vi "ColorizeREPL.vi"(0 "Data In":T1={"VISA Refnum in"="", "Python Code"="Hi"}, 2 "refs":cluster{"Code":refnum<vi>, "Panel":refnum<vi>}, 4 "Add Spaces?":bool) -> (7 "Data out":T1={"VISA Refnum in"="", "Python Code"="Hi"})   [LabVIEW 2016]
uses:
  <vilib>/Utility/miscctls.llb/LVSelectionTypeDef.ctl
  uPythonX/PythonData.ctl
  uPythonX/uPythonX.xctl
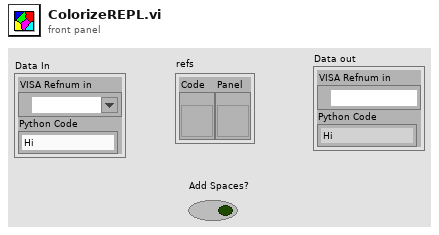
[diagram p1: front panel]
types:
  T1 = typedef "uPythonX.xctl/PythonData.ctl" = cluster{"VISA Refnum in":refnum<visa-resource-name>, "Python Code":string}
  T2 = typedef "LVSelectionTypeDef.ctl" = cluster{"Selection Start":u32, "Selection End":u32}
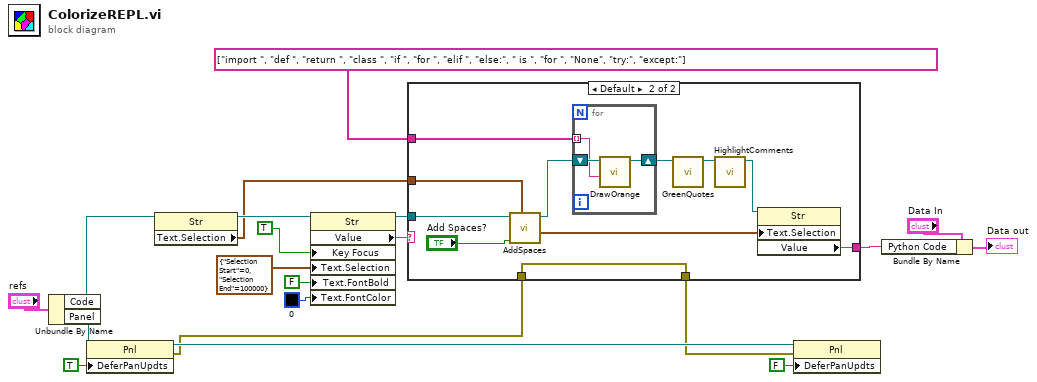
[diagram p0: block diagram]
diagram:
  n1 = Unbundle By Name("refs") -> ("Code"=w3:refnum<vi>, "Panel"=w4:refnum<vi>)
  n2 = property class="Pnl"(reference=w4, "DeferPanUpdts"=TRUE ("Defer Panel Updates")) -> (reference out=w6:refnum<vi>, error out=w1:errorcluster)  [unwired: 1 in]
  n3 = property on="Property Node" class="Str"(reference=w3) -> (reference out=w16:refnum<vi>, "Text.Selection"=w15:T2)  [unwired: 1 in, 1 out]
  n4 = property on="Property Node" class="Str"(reference=w16, "Key Focus"=TRUE, "Text.Selection"=T2 {"Selection Start"=0, "Selection End"=100000}, "Text.FontBold"=FALSE ("Text.Font:Bold"), "Text.FontColor"=u32 0) -> (reference out=w14:refnum<vi>, "Value"=w13:string)  [unwired: 1 in, 1 out]
  n5 = case shown="Default" w13 {
    selector: w13 -> [w22 _]
    tunnel: w14 -> [_ w27]
    tunnel: w15 -> [_ w32]
    tunnel: [w22 w30] -> w10
    tunnel: string[] ["import ", "def ", "return ", "class ", "if ", "for ", "elif ", "else:", " is ", "for ", "None", "try:", "except:"] -> [_ w25]
    tunnel: [w21 w23] -> w2
    tunnel: w1 -> [w21 w23]
    frame "" {
    }
    frame Default {
      n6 = call "AddSpaces.vi"("Text.Selection"=w32, "Add Spaces?"="Add Spaces?", "String in"=w27) -> ("Cursor"=w29:cluster{u32, u32}, "String out"=w26:refnum<vi>)  [unwired: 7 in]
      n7 = for {
        shift-right: [w35] -> w33
        shift-left: w26 -> [w36]
        tunnel: w25 -> [w34] mode=indexing
        n8 = call "DrawOrange.vi"("Expression"=w34, "String in"=w36) -> ("String out"=w35:refnum<vi>)  [unwired: 9 in]
      }
      n9 = call "GreenQuotes.vi"("String in"=w33) -> ("String out"=w31:refnum<vi>)  [unwired: 10 in]
      n10 = call "HighlightComments.vi"("String in"=w31) -> ("String out"=w28:refnum<vi>)  [unwired: 10 in]
      n11 = property on="Property Node" class="Str"(reference=w28, "Text.Selection"=w29) -> ("Value"=w30:string)  [unwired: 1 in, 2 out]
    }
  }
  n12 = property class="Pnl"(reference=w6, error in=w2, "DeferPanUpdts"=FALSE ("Defer Panel Updates")) -> ()  [unwired: 2 out]
  n13 = Bundle By Name(cluster="Data In", "Python Code"=w10) -> (→"Data out":T1)
